vi "test_OneSessTwoPinOneInstrTwoSiteReservation_CallNiDigitalGetConnections1Pin1Connection_ReturnsOneConnection.vi"(8 "error in":errorcluster) -> (0 "error out":errorcluster, 2 "result":string, 3 "pass":bool)   [LabVIEW 2020, in "MeasurementServerTests.lvlib"]
uses:
  MeasurementServerTests.lvlib
  Runtime/Clients/Session Management V1/Session Reservation/Connection.ctl
  Runtime/Sessions/niDigital Sessions/Connection with Session.ctl
  03fc85e1-696b-4ece-a78b-f41470766ac0.vi
  d597c107-a9cb-4c8e-b2d9-e6157ee92f08.vi
  <vilib>/AdvancedString/1D String Array to Delimited String.vi
  d597c107-a9cb-4c8e-b2d9-e6157ee92f08.vi/94283ac5-2298-4b3a-b57d-7be67da3787d.vi
  d597c107-a9cb-4c8e-b2d9-e6157ee92f08.vi/f7d9c9cb-0251-4d67-81cb-70e1b0e8b69f.vi
  Runtime/Sessions/niDigital Sessions/Get Connections - 1Pin 1Conn.vi
  <vilib>/JDP Science/JSONtext/Variant to JSON Text.vi
  <vilib>/JDP Science/JSONtext/LVClass Serializer/JSONtext LVClass Serializer.lvclass
  Runtime/Clients/Session Management V1/Session Reservation/Session Reservation.lvclass
  Runtime/Sessions/niDigital Sessions/Plug-In SDK niDigital Sessions.lvlib
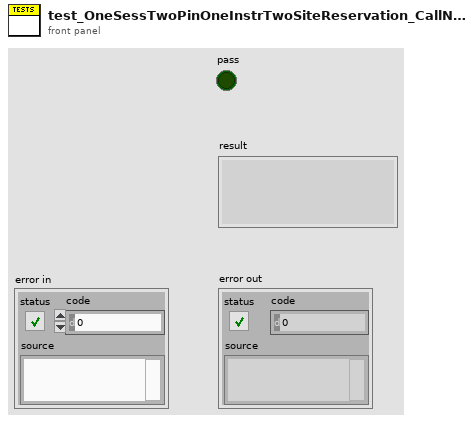
[diagram p1: front panel]
types:
  T1 = typedef "Plug-In SDK niDigital Sessions.lvlib/Connection with Session.ctl" = cluster{"connection":T2, "session":refnum<k15>}
  T2 = typedef "NI Session Management V1 Client.lvlib/Session Reservation.lvclass/Connection.ctl" = cluster{"pin or relay name":string, "site":i32, "instrument type id":string, "channel":string}
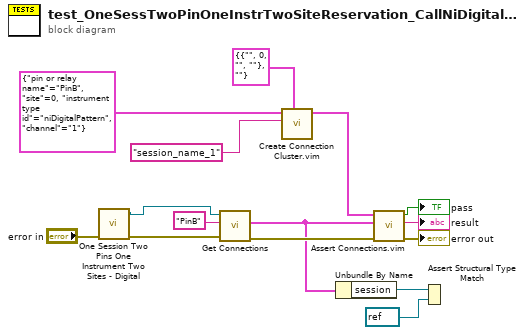
[diagram p0: block diagram]
diagram:
  n1 = call "One Session Two Pins One Instrument Two Sites - Digital.vi"("error in"="error in") -> ("error out"=w4:errorcluster, "session reservation out"=w5:refnum<class "Session Reservation.lvclass">)  [unwired: 9 in]
  n2 = call-poly "Get Connections.vi"("error in"=w4, "pin or relay name"="PinB", "session reservation in"=w5) -> ("error out"=w3:errorcluster, "connection"=w1:T1)  [unwired: 6 in, 1 out]
  n3 = call "Create Connection Cluster.vim"("connection type"=T1 {"connection"={"pin or relay name"="", "site"=0, "instrument type id"="", "channel"=""}, "session"=""} ("connection with session"), "session in"="session_name_1", "hardware independent connection in"=T2 {"pin or relay name"="PinB", "site"=0, "instrument type id"="niDigitalPattern", "channel"="1"} ("connection")) -> ("connection out"=w13:T1)  [unwired: 8 in]
  n4 = Unbundle By Name(w1) -> ("session"=w7:refnum<k15>)
  n5 = call "Assert Connections.vim"("error in"=w3, "actual connections"=w1, "expected connections"=w13) -> ("error out"=→"error out":errorcluster, "result"=→"result":string, "pass"=→"pass":bool)  [unwired: 6 in]
  n6 = Assert Structural Type Match(0:refnum<k15> refnum ("session"), 1:w7) -> ()
